vi "Validate Project Path.vi"(11 "error in (no error)":errorcluster) -> (4 "Valid Path?":bool, 15 "error out":errorcluster)   [LabVIEW 2021, in "Packager Helpers.lvlib"]
uses:
  Packager Helpers.lvlib
  Dictionary/Dictionary.lvlib
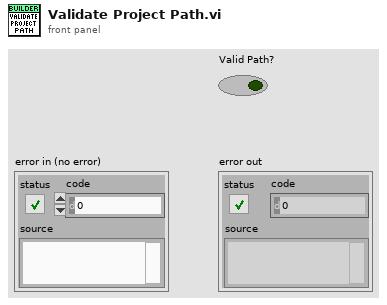
[diagram p1: front panel]
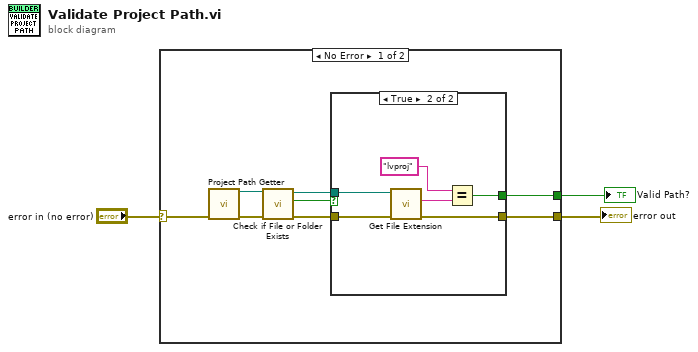
[diagram p0: block diagram]
diagram:
  n1 = case shown="No Error" "error in (no error)" {
    selector: "error in (no error)" -> [w11 w20]
    tunnel: [w5 _] -> w2
    tunnel: [w4 w20] -> w1
    frame No Error {
      n2 = call "Project Path Getter.vi"("error in (no error)"=w11) -> ("Path"=w9:path, "error out"=w10:errorcluster)  [unwired: 13 in]
      n3 = call <vilib>:"Check if File or Folder Exists.vi"("error in (no error)"=w10, "path"=w9) -> ("error out"=w7:errorcluster, "file or folder exists?"=w8:bool, "dup path"=w6:path)  [unwired: 7 in]
      n4 = case shown="True" w8 {
        selector: w8 -> [w13 _]
        tunnel: w7 -> [w12 w19]
        tunnel: w6 -> [_ w18]
        tunnel: [w13 w15] -> w5
        tunnel: [w12 w14] -> w4
        frame False {
        }
        frame True {
          n5 = call <vilib>:"Get File Extension.vi"("error in (no error)"=w19, "file"=w18) -> ("error out"=w14:errorcluster, "lowercase file extension"=w17:string)  [unwired: 5 in, 3 out]
          n6 = Equal?(x="lvproj", y=w17) -> (x = y?=w15:bool)
        }
      }
    }
    frame Error {
    }
  }
  "error out" <- w1
  "Valid Path?" <- w2
